vi "Write auto.vi"(8 "error in (no error)":errorcluster, 10 "auto":bool, 11 "Change AutoCycle Params MSG in":refnum<class "Change AutoCycle Params MSG.lvclass">) -> (0 "error out":errorcluster, 3 "Change AutoCycle Params MSG out":refnum<class "Change AutoCycle Params MSG.lvclass">)   [LabVIEW 2016, in "Change AutoCycle Params MSG.lvclass"]
uses:
  Change AutoCycle Params MSG.lvclass
  Change AutoCycle Params MSG.lvclass/Change AutoCycle Params MSG.ctl
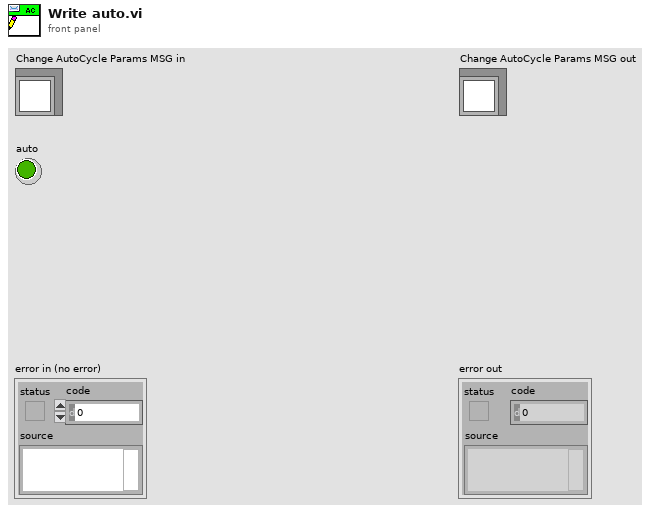
[diagram p1: front panel]
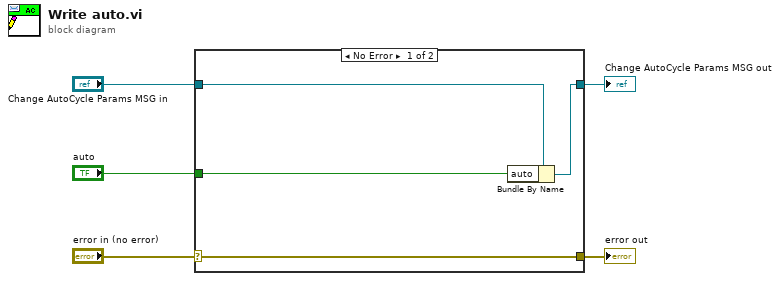
[diagram p0: block diagram]
diagram:
  n1 = case shown="No Error" "error in (no error)" {
    selector: "error in (no error)" -> [w9 w10]
    tunnel: [w9 w10] -> w4
    tunnel: [w7 w11] -> w2
    tunnel: "Change AutoCycle Params MSG in" -> [w8 w11]
    tunnel: "auto" -> [w6 _]
    frame No Error {
      n2 = Bundle By Name(cluster=w8, "auto"=w6) -> (w7:refnum<class "Change AutoCycle Params MSG.lvclass">)
    }
    frame Error {
    }
  }
  "error out" <- w4
  "Change AutoCycle Params MSG out" <- w2
